vi "Batch_ListReposBranches.vi"(8 "error in (no error)":errorcluster, 11 "CommandLine":string[](array[string])) -> (0 "error out":errorcluster, 2 "test details":string, 3 "output to action":string)   [LabVIEW 2017]
uses:
  _lvcicd/_lvcicd_support_2017.lvlib
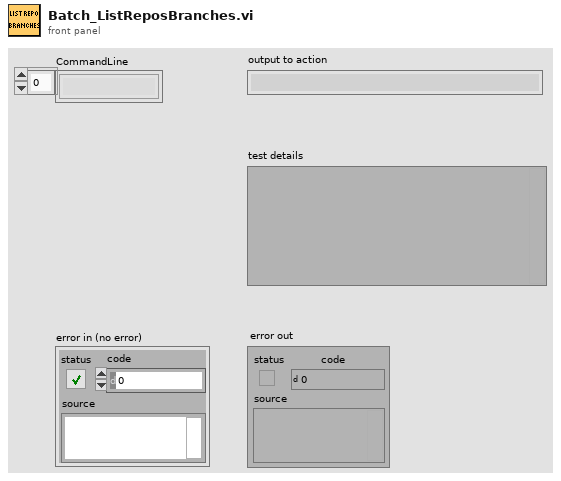
[diagram p1: front panel]
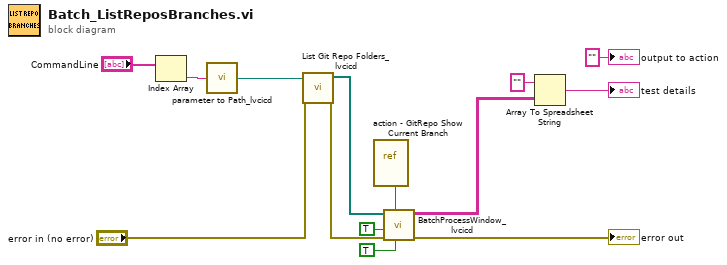
[diagram p0: block diagram]
diagram:
  n1 = Index Array(array="CommandLine") -> (element=w3:string)  [unwired: 1 in]
  n2 = call "parameter to Path_lvcicd.vi"("String"=w3) -> ("Path"=w2:path)
  n3 = call "List Git Repo Folders_lvcicd.vi"("error in (no error)"="error in (no error)", "path"=w2) -> ("error out"=w7:errorcluster, "Repo Folders"=w13:path[])  [unwired: 8 in]
  n4 = vi-ref "action - GitRepo Show Current Branch.vi"() -> (w8:refnum<vi>)
  n5 = call "BatchProcessWindow_lvcicd.vi"("FP(T)"=TRUE, "VI Refnum"=w8, "error in (no error)"=w7, "silence mode(F)"=TRUE, "paths"=w13) -> ("error out"=→"error out":errorcluster, "Array"=w12:string[][])  [unwired: 5 in]
  n6 = Array To Spreadsheet String(array=w12, 3:"" ("format string")) -> (spreadsheet string=→"test details":string)  [unwired: 1 in]
  "output to action" <- "" ("output to action")
